vi "start_stream.vi"(6 "Period [ms]":i32=500 min=1 max=60000, 8 "error in (no error)":errorcluster, 11 "Handle In":i32) -> (0 "error out":errorcluster, 1 "NumReadAddresses":i32, 2 "ScansPerRead Out":i32, 3 "Handle Out":i32)   [LabVIEW 2025, in "LabJackEKG.lvlib"]
uses:
  LabJackEKG.lvlib
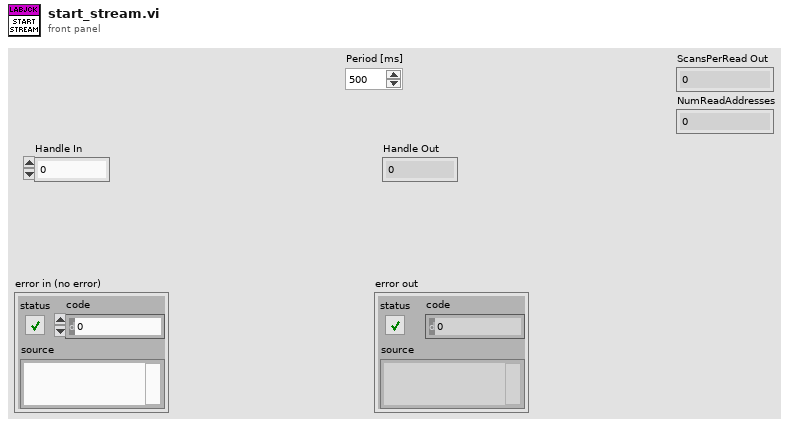
[diagram p1: front panel]
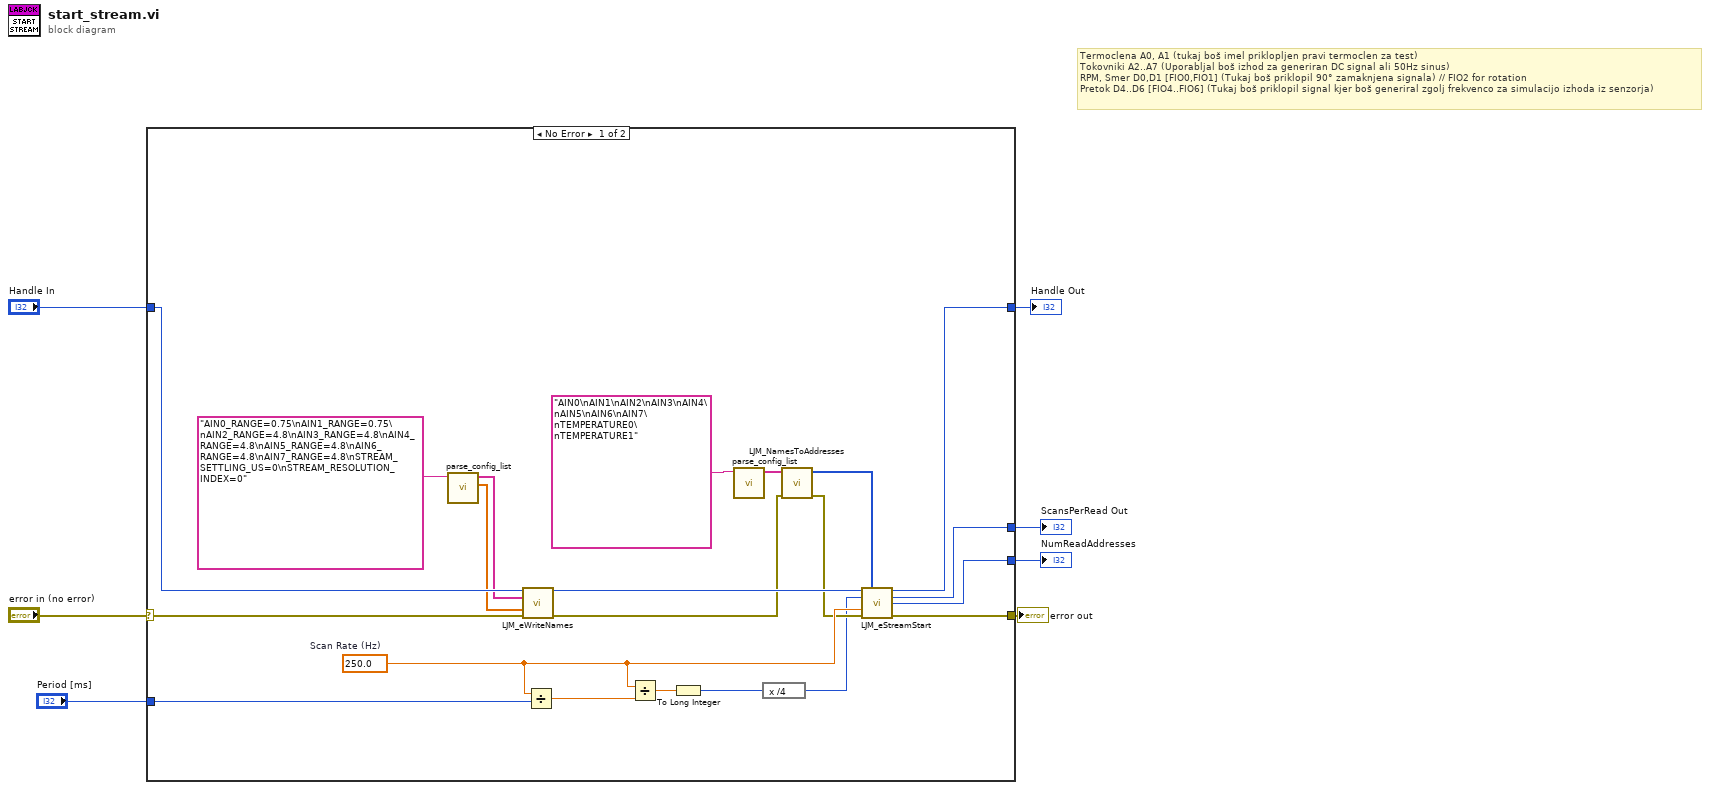
[diagram p0: block diagram]
diagram:
  # "Termoclena A0, A1 (tukaj boš imel priklopljen pravi termoclen za test)\nTokovniki A2..A7 (Uporabljal boš izhod za generiran DC signal ali 50Hz sinus)\nRPM, Smer D0,D1 [FIO0,FIO1] (Tukaj boš priklopil 90° zamaknjena signala) // FIO2 for rotation\nPretok D4..D6 [FIO4..FIO6] (Tukaj boš priklopil signal kjer boš generiral zgolj frekvenco za simulacijo izhoda iz senzorja)"
  n1 = case shown="No Error" "error in (no error)" {
    selector: "error in (no error)" -> [w28 w30]
    tunnel: [w23 w29] -> w7
    tunnel: "Handle In" -> [w27 w29]
    tunnel: [w24 w30] -> w4
    tunnel: [w21 _] -> w3
    tunnel: [w20 _] -> w2
    tunnel: "Period [ms]" -> [w19 _]
    frame No Error {
      w18 = 250.0  # Scan Rate (Hz)
      n2 = call "parse_config_list.vi"("String"="AIN0_RANGE=0.75\nAIN1_RANGE=0.75\nAIN2_RANGE=4.8\nAIN3_RANGE=4.8\nAIN4_RANGE=4.8\nAIN5_RANGE=4.8\nAIN6_RANGE=4.8\nAIN7_RANGE=4.8\nSTREAM_SETTLING_US=0\nSTREAM_RESOLUTION_INDEX=0") -> ("Values"=w14:dbl[], "Names"=w15:string[])  [unwired: 9 in]
      n3 = call <vilib>:"LJM_eWriteNames.vi"("Handle In"=w27, "aNames"=w15, "aValuesIn"=w14, "error in"=w28) -> ("Handle Out"=w25:i32, "error out"=w10:errorcluster)  [unwired: 9 in, 1 out]
      n4 = Divide(x=w18, y=w19) -> (x/y=w17:dbl)
      n5 = Divide(x=w18, y=w17) -> (x/y=w26:dbl)
      n6 = To Long Integer(number=w26) -> (32bit integer=w22:i32)
      n7 = call "parse_config_list.vi"("String"="AIN0\nAIN1\nAIN2\nAIN3\nAIN4\nAIN5\nAIN6\nAIN7\nTEMPERATURE0\nTEMPERATURE1") -> ("Names"=w12:string[])  [unwired: 9 in, 1 out]
      n8 = expression code="x /4"(w22) -> (w8:i32)
      n9 = call <vilib>:"LJM_NamesToAddresses.vi"("error in"=w10, "aNames"=w12) -> ("error out"=w9:errorcluster, "aAddresses"=w11:i32[])  [unwired: 7 in, 1 out]
      n10 = call <vilib>:"LJM_eStreamStart.vi"("Handle In"=w25, "aScanList"=w11, "ScansPerRead"=w8, "ScanRate"=w18, "error in"=w9) -> ("Handle Out"=w23:i32, "ScansPerRead Out"=w20:i32, "NumReadAddresses"=w21:i32, "error out"=w24:errorcluster)  [unwired: 5 in, 2 out]
    }
    frame Error {
    }
  }
  "error out" <- w4
  "Handle Out" <- w7
  "ScansPerRead Out" <- w2
  "NumReadAddresses" <- w3
